vi "mailids.vi"() -> ()   [LabVIEW 2018]
panel:
  out "Numeric":dbl
  in  "String 3":string
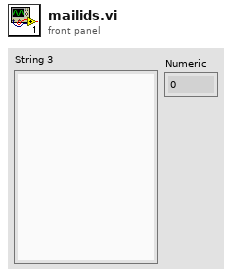
[diagram p1: front panel]
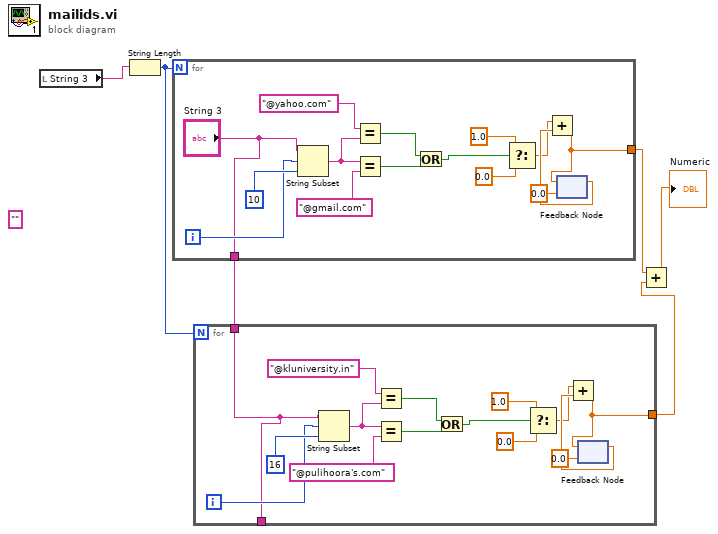
[diagram p0: block diagram]
diagram:
  (unwired) "" ("regular expression")
  n1 = local read "String 3"() -> (w6:string)
  n2 = String Length(string=w6) -> (length=w4:i32)
  n3 = for {
    N: w4 -> [_]
    tunnel: [w14] -> w2
    tunnel: ["String 3"] -> w5
    i -> [w13]
    n4 = String Subset(string="String 3", offset (0)=w13, length (rest)=10 ("length (rest)")) -> (substring=w12:string)
    n5 = Equal?(x="@yahoo.com" ("y"), y=w12) -> (x = y?=w10:bool)
    n6 = Equal?(x=w12, y="@gmail.com") -> (x = y?=w9:bool)
    n7 = Or(x=w10, y=w9) -> (x .or. y?=w8:bool)
    n8 = Select(t=1.0, s=w8, f=0.0) -> (s? t:f=w15:dbl)
    n9 = feedback #1(0.0) -> (w19:dbl)
    n10 = Add(x=w15, y=w19) -> (x+y=w14:dbl)
    n11 = feedback-in #1(w14) -> ()
  }
  n12 = for {
    N: w4 -> [_]
    tunnel: [w29] -> w3
    tunnel: [w22] -> _
    tunnel: w5 -> [w22]
    i -> [w28]
    n13 = String Subset(string=w22, offset (0)=w28, length (rest)=16 ("length (rest)")) -> (substring=w27:string)
    n14 = Equal?(x="@kluniversity.in" ("y"), y=w27) -> (x = y?=w25:bool)
    n15 = Equal?(x=w27, y="@pulihoora's.com") -> (x = y?=w24:bool)
    n16 = Or(x=w25, y=w24) -> (x .or. y?=w23:bool)
    n17 = Select(t=1.0, s=w23, f=0.0) -> (s? t:f=w30:dbl)
    n18 = feedback #2(0.0) -> (w34:dbl)
    n19 = Add(x=w30, y=w34) -> (x+y=w29:dbl)
    n20 = feedback-in #2(w29) -> ()
  }
  n21 = Add(x=w2, y=w3) -> (x+y=→"Numeric":dbl)
